vi "Get Request Type.vi"(8 "error in (no error)":errorcluster, 11 "GetSceneItemID in":refnum<class "GetSceneItemID.lvclass">) -> (0 "error out":errorcluster, 2 "Request Type":string, 3 "GetSceneItemID out":refnum<class "GetSceneItemID.lvclass">)   [LabVIEW 2020, in "obs-websocket.lvlib" / "GetSceneItemID.lvclass"]
uses:
  GetSceneItemID.lvclass
  GetSceneItemID.lvclass/GetSceneItemID.ctl
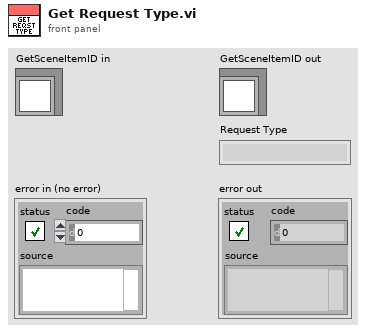
[diagram p1: front panel]
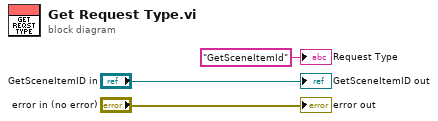
[diagram p0: block diagram]
diagram:
  "error out" <- "error in (no error)"
  "GetSceneItemID out" <- "GetSceneItemID in"
  "Request Type" <- "GetSceneItemId" ("Request Type")
